vi "Command Runner.vi"(10 "Data":variant, 11 "Command Name":string) -> ()   [LabVIEW 2018]
uses:
  AutonBuilder/Typedef/String Commands.ctl
  Auton Kill Switch.vi
  Drive/Pure Pursuit/Typedef/Pure Pursuit Telemetry.ctl
  Drive/Pure Pursuit/Typedef/Path Point.ctl
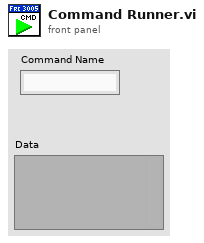
[diagram p1: front panel]
types:
  T1 = typedef "String Commands.ctl" = string
  T2 = typedef "Pure Pursuit.lvlib/Pure Pursuit Telemetry.ctl" = cluster{"Target Point":T3, "Close Point":T3, "Curvature":dbl, "index out":i32}
  T3 = typedef "Pure Pursuit.lvlib/Path Point.ctl" = cluster{"x":dbl, "y":dbl, "heading":dbl, "curvature":dbl, "total distance":dbl, "velocity expected":dbl}
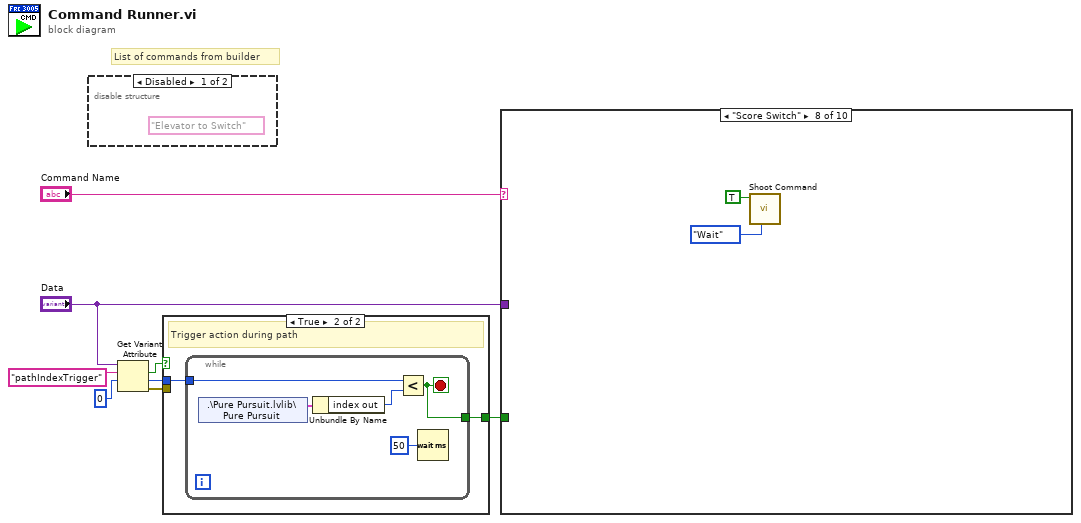
[diagram p0: block diagram]
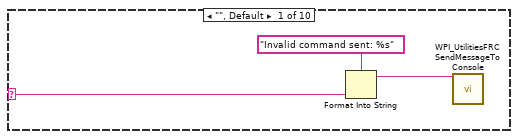
[diagram p4: hidden frame]
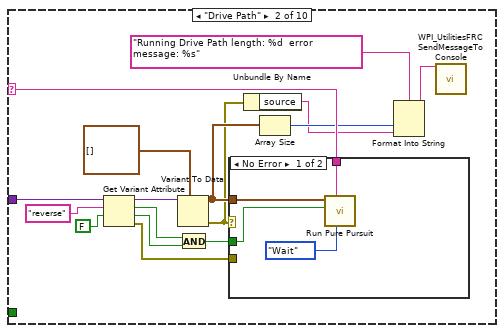
[diagram p5: hidden frame]
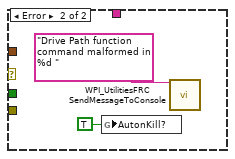
[diagram p6: hidden frame]
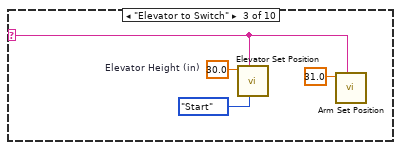
[diagram p7: hidden frame]
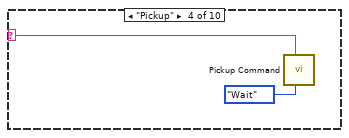
[diagram p8: hidden frame]
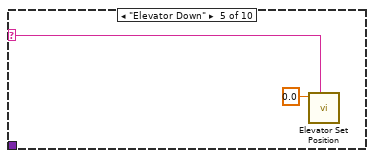
[diagram p9: hidden frame]
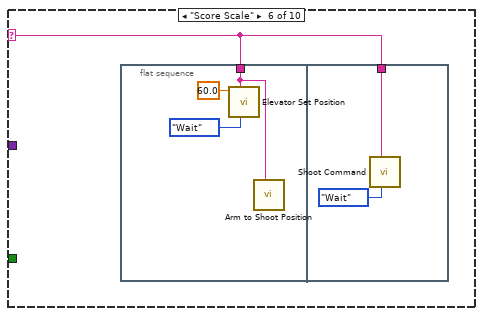
[diagram p10: hidden frame]
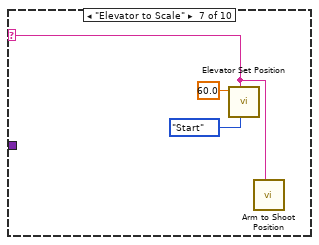
[diagram p11: hidden frame]
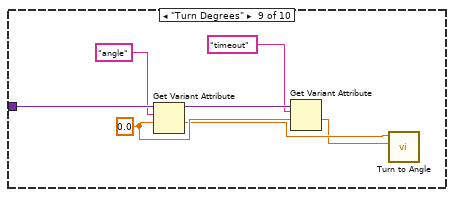
[diagram p12: hidden frame]
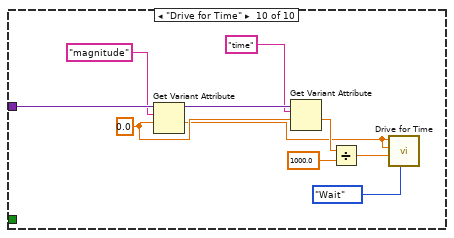
[diagram p13: hidden frame]
diagram:
  # "List of commands from builder"
  n1 = disable-structure shown="Disabled" {
    frame Disabled {
      (unwired) T1 "Elevator to Switch" ("Other Commands")
    }
    frame Enabled {
    }
  }
  n2 = Get Variant Attribute(Variant="Data", name="pathIndexTrigger", default value (empty Variant)=0 ("index out")) -> (found=w3:bool, value=w4:i32, error out=w5:errorcluster)  [unwired: 1 in, 1 out]
  n3 = case shown="True" w3 {
    tunnel: w5 -> [_ _]
    tunnel: w4 -> [_ w9]
    tunnel: [_ w10] -> w2
    frame False {
    }
    frame True {
      # "Trigger action during path"
      n4 = while {
        tunnel: w9 -> [w14]
        tunnel: [w11] -> w10
        stop <- w11 stop-if-true
        n5 = shared-variable ".\\Pure Pursuit.lvlib\\Pure Pursuit"() -> (w15:T2)  [unwired: 1 in, 1 out]
        n6 = Unbundle By Name(w15) -> ("index out"=w13:i32)
        n7 = Less?(x=w14, y=w13) -> (x < y?=w11:bool)
        n8 = Wait (ms)(milliseconds to wait=u32 50) -> ()  [unwired: 1 out]
      }
    }
  }
  n9 = case shown="\"Score Switch\"" "Command Name" {
    selector: "Command Name" -> [w18 w34 w41 w45 w47 w49 w57 _ _ _]
    tunnel: "Data" -> [_ w33 _ _ _ _ _ _ w66 w76]
    tunnel: w2 -> [_ _ _ _ _ _ _ _ _ _]
    frame "", Default {
      n10 = Format Into String(format string="Invalid command sent: %s", w18) -> (resulting string=w17:string)  [unwired: 2 in, 1 out]
      n11 = call <vilib>:"WPI_UtilitiesFRC SendMessageToConsole.vi"("Message"=w17) -> ()  [unwired: 14 in, 1 out]
    }
    frame "Drive Path" {
      n12 = Get Variant Attribute(Variant=w33, name="reverse" ("Current Command.Command Name"), default value (empty Variant)=FALSE) -> (duplicate Variant=w25:variant, found=w22:bool, value=w21:bool, error out=w23:errorcluster)  [unwired: 1 in]
      n13 = Variant To Data(type=cluster{dbl, "interpolation value":dbl}[] [] ("Path"), Variant=w25) -> (data=w29:cluster{dbl, "interpolation value":dbl}[], error out=w27:errorcluster)  [unwired: 1 in]
      n14 = And(x=w22, y=w21) -> (x .and. y?=w20:bool)
      n15 = case shown="No Error" w27 {
        tunnel: w34 -> [w38 _]
        tunnel: w29 -> [w37 _]
        tunnel: w23 -> [_ _]
        tunnel: w20 -> [w35 _]
        frame No Error {
          n16 = call "Run Pure Pursuit.vi"("Synchronication"=enum16{"Start", "Wait"}."Wait", "Description"=w38, "Reverse? (F)"=w35, "Path"=w37) -> ()  [unwired: 7 in, 1 out]
        }
        frame Error {
          n17 = global write "Auton Kill Switch.vi" "AutonKill?"(TRUE ("AutonKill?")) -> ()
          n18 = call <vilib>:"WPI_UtilitiesFRC SendMessageToConsole.vi"("Message"="Drive Path function command malformed in %d ") -> ()  [unwired: 14 in, 1 out]
        }
      }
      n19 = Unbundle By Name(w27) -> ("source"=w26:string)
      n20 = Array Size(array=w29) -> (size(s)=w28:i32)
      n21 = Format Into String(format string="Running Drive Path length: %d  error message: %s", w28, w26) -> (resulting string=w31:string)  [unwired: 2 in, 1 out]
      n22 = call <vilib>:"WPI_UtilitiesFRC SendMessageToConsole.vi"("Message"=w31) -> ()  [unwired: 14 in, 1 out]
    }
    frame "Elevator to Switch" {
      w44 = 30.0  # Elevator Height (in)
      n23 = call "Elevator Set Position.vi"("Synchronization"=enum16{"Start", "Wait"}."Start", "Description"=w41, "Setpoint"=w44) -> ()  [unwired: 8 in, 1 out]
      n24 = call "Arm Set Position.vi"("Description"=w41, "Setpoint"=31.0) -> ()  [unwired: 9 in, 1 out]
    }
    frame "Pickup" {
      n25 = call "Pickup Command.vi"("Synchronization"=enum16{"Start", "Wait"}."Wait", "Description"=w45) -> ()  [unwired: 9 in, 1 out]
    }
    frame "Elevator Down" {
      n26 = call "Elevator Set Position.vi"("Description"=w47, "Setpoint"=0.0) -> ()  [unwired: 9 in, 1 out]
    }
    frame "Score Scale" {
      n27 = flat-sequence {
        tunnel: w49 -> [w50]
        tunnel: w49 -> [w53]
        frame #0 {
          n28 = call "Elevator Set Position.vi"("Synchronization"=enum16{"Start", "Wait"}."Wait", "Description"=w50, "Setpoint"=60.0) -> ()  [unwired: 8 in, 1 out]
          n29 = call "Arm to Shoot Position.vi"("Description"=w50) -> ()  [unwired: 10 in, 1 out]
        }
        frame #1 {
          n30 = call "Shoot Command.vi"("Synchronization"=enum16{"Start", "Wait"}."Wait", "Description"=w53) -> ()  [unwired: 9 in, 1 out]
        }
      }
    }
    frame "Elevator to Scale" {
      n31 = call "Elevator Set Position.vi"("Synchronization"=enum16{"Start", "Wait"}."Start", "Description"=w57, "Setpoint"=60.0) -> ()  [unwired: 8 in, 1 out]
      n32 = call "Arm to Shoot Position.vi"("Description"=w57) -> ()  [unwired: 10 in, 1 out]
    }
    frame "Score Switch" {
      n33 = call "Shoot Command.vi"("Synchronization"=enum16{"Start", "Wait"}."Wait", "Soft Shot?"=TRUE) -> ()  [unwired: 9 in, 1 out]
    }
    frame "Turn Degrees" {
      w62 = 0.0
      n34 = Get Variant Attribute(Variant=w66, name="angle", default value (empty Variant)=w62) -> (duplicate Variant=w64:variant, value=w61:dbl)  [unwired: 1 in, 2 out]
      n35 = Get Variant Attribute(Variant=w64, name="timeout", default value (empty Variant)=w62) -> (value=w60:dbl)  [unwired: 1 in, 3 out]
      n36 = call "Turn to Angle.vi"("Duration"=w60, "Setpoint"=w61) -> ()  [unwired: 9 in, 1 out]
    }
    frame "Drive for Time" {
      w72 = 0.0
      n37 = Get Variant Attribute(Variant=w76, name="magnitude", default value (empty Variant)=w72) -> (duplicate Variant=w74:variant, value=w69:dbl)  [unwired: 1 in, 2 out]
      n38 = Get Variant Attribute(Variant=w74, name="time", default value (empty Variant)=w72) -> (value=w71:dbl)  [unwired: 1 in, 3 out]
      n39 = Divide(x=w71, y=1000.0) -> (x/y=w68:dbl)
      n40 = call "Drive for Time.vi"("Synchronization"=enum16{"Start", "Wait"}."Wait", "Seconds"=w68, "Right Speed"=w69, "Left Speed"=w69) -> ()  [unwired: 6 in, 2 out]
    }
  }
